vi "Get Text Rect.vi"(0 "alignment(left, top)":T1, 1 "desired font(Application)":T2(ring), 2 "origin(0,0)":cluster{"horizontal":i16, "vertical":i16}, 3 "text":string, 4 "text orientation":T3(ring), 5 "[user-specified font]":T4) -> (6 "rect":T5)   [LabVIEW 2021, in "Picture Pixel Fonts.lvlib"]
uses:
  <vilib>/LabVIEW Icon API/Pixel Fonts/Picture Pixel Fonts.lvlib
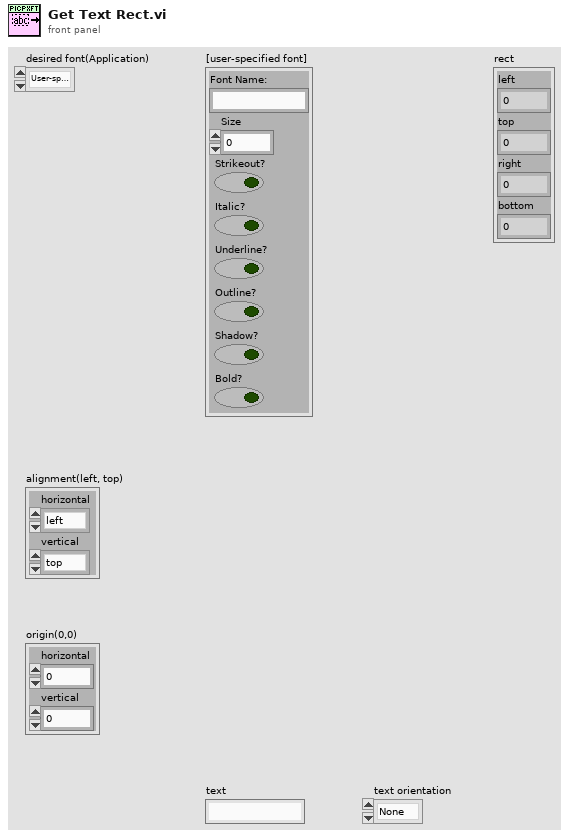
[diagram p1: front panel]
types:
  T1 = cluster{"horizontal":enum16{"left", "center", "right"}, "vertical":enum16{"top", "center", "bottom"}}
  T2 = enum16{"User-specified Font", "Application Font", "System Font", "Dialog Font"}
  T3 = enum16{"None", "Stacked", "Clockwise", "Counterclockwise"}
  T4 = cluster{"Font Name:":string, "Size":i16, "Strikeout?":bool, "Italic?":bool, "Underline?":bool, "Outline?":bool, "Shadow?":bool, "Bold?":bool}
  T5 = cluster{"left":i16, "top":i16, "right":i16, "bottom":i16}
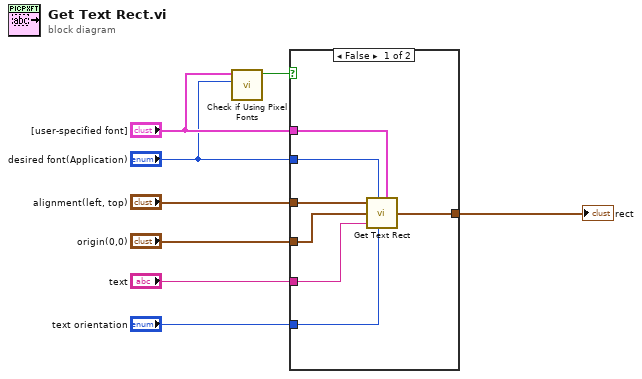
[diagram p0: block diagram]
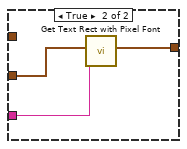
[diagram p2: hidden frame]
diagram:
  n1 = call <vilib>:"Check if Using Pixel Fonts.vi"("desired font(Application)"="desired font(Application)", "[user-specified font]"="[user-specified font]") -> ("use_pixel_fonts"=w1:bool)  [unwired: 9 in]
  n2 = case shown="False" w1 {
    tunnel: [w15 w17] -> w8
    tunnel: "text orientation" -> [w14 _]
    tunnel: "text" -> [w13 w16]
    tunnel: "origin(0,0)" -> [w12 w18]
    tunnel: "alignment(left, top)" -> [w11 _]
    tunnel: "[user-specified font]" -> [w10 _]
    tunnel: "desired font(Application)" -> [w9 _]
    frame False {
      n3 = call <vilib>:"Get Text Rect.vi"("alignment(left, top)"=w11, "desired font(Application)"=w9, "origin(0,0)"=w12, "text"=w13, "text orientation"=w14, "[user-specified font]"=w10) -> ("rect"=w15:T5)  [unwired: 3 in]
    }
    frame True {
      n4 = call <vilib>:"Get Text Rect with Pixel Font.vi"("string"=w16, "origin"=w18) -> ("Rectangle out"=w17:T5)  [unwired: 9 in]
    }
  }
  "rect" <- w8
